vi "File.Excel, Concatinate Excel Files In a Folder.vi"(7 "Pattern":string="*.xlsx", 8 "error in (no error)":errorcluster, 10 "Output Name":string="Concat Data", 11 "Folder":path) -> (0 "error out":errorcluster)   [LabVIEW 2019]
uses:
  <vilib>/KATE/Files/File Utils.lvlib
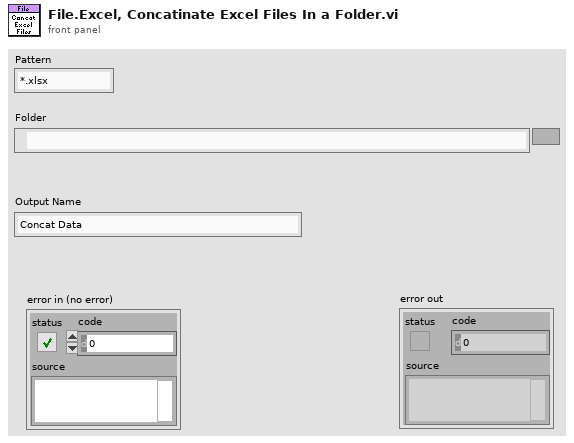
[diagram p1: front panel]
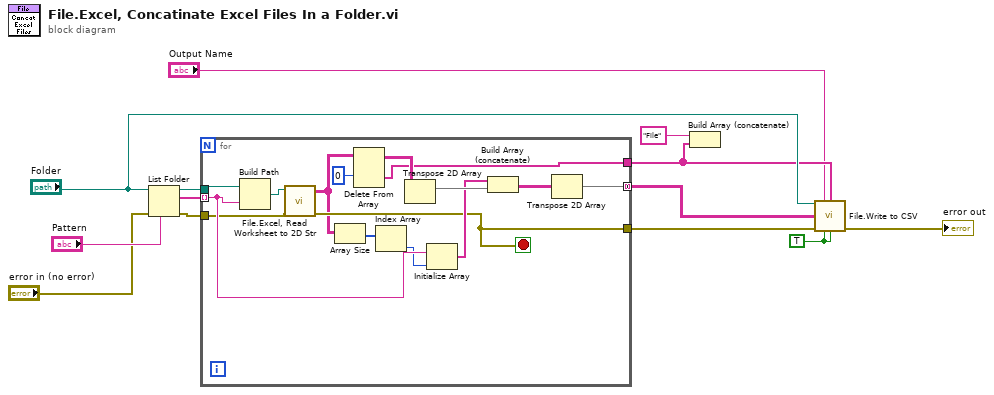
[diagram p0: block diagram]
diagram:
  w4 = TRUE ("Append Time to Filename")
  n1 = List Folder(path="Folder", pattern="Pattern", error in="error in (no error)") -> (path out=w12:path, filenames=w5:string[], error out=w1:errorcluster)  [unwired: 1 in, 1 out]
  n2 = for {
    tunnel: w12 -> [w24]
    tunnel: [w14] -> w9
    tunnel: [w20] -> w8
    tunnel: w5 -> [w23] mode=indexing
    tunnel: [w25] -> w3 mode=concatenating
    tunnel: w1 -> [w21]
    stop <- w20 stop-if-true
    n3 = Build Path(base path=w24, name or relative path=w23) -> (appended path=w22:path)
    n4 = call "File.Excel, Read Worksheet to 2D Str.vi"("error in (no error)"=w21, "Excel File Path"=w22) -> ("error out"=w20:errorcluster, "Data"=w17:string[][])  [unwired: 8 in]
    n5 = Array Size(array=w17) -> (size(s)=w19:i32[])
    n6 = Delete From Array(array=w17, index (row)=0) -> (deleted portion=w14:string[], array with subset deleted=w15:string[][])  [unwired: 2 in]
    n7 = Index Array(array=w19) -> (element=w18:i32)  [unwired: 1 in]
    n8 = Transpose 2D Array(2D array=w15) -> (transposed array=w28:string[][])
    n9 = Initialize Array(w23, w18) -> (w27:string[])
    n10 = Build Array (concatenate)(w27, w28) -> (w26:string[][])
    n11 = Transpose 2D Array(2D array=w26) -> (transposed array=w25:string[][])
  }
  n12 = Build Array (concatenate)("File", w9) -> ()  [unwired: 1 out]
  n13 = call <vilib>:"File.Write to CSV.vi"("Folder"="Folder", "FileRootName"="Output Name", "Header"=w9, "2D"=w3, "error in"=w8, "Append Time to Filename"=w4, "Append Date to Filename"=w4) -> ("error out"=→"error out":errorcluster)  [unwired: 7 in, 1 out]
